vi "readModbusRxData.vi"(8 "error in (no error)":errorcluster, 9 "Timeout (ms)":i32, 10 "ModbusBuffer in":refnum<class "ModbusBuffer.lvclass">, 11 "FPGA in":refnum<class "FPGA.lvclass">) -> (0 "error out":errorcluster, 1 "Elements Remaining":u32, 2 "ModbusBuffer out":refnum<class "ModbusBuffer.lvclass">, 3 "FPGA out":refnum<class "FPGA.lvclass">)   [LabVIEW 2016, in "FPGA.lvclass"]
uses:
  FPGA.lvclass
  Common_RT_Modbus/ModbusBuffer/ModbusBuffer.lvclass
  FPGA.lvclass/FPGA.ctl
  Common_RT_Modbus/ModbusBuffer/ModbusBuffer.lvclass/ModbusBuffer.ctl
  <vilib>/Utility/error.llb/Error Cluster From Error Code.vi
  <vilib>/rvi/errors/niLvFpgaAdjustHostInterfaceError.vi
  <vilib>/rvi/interface/nirviMethod/nirviMethod.xnode
  <vilib>/rvi/errors/niLvFpgaMergeErrorWithErrorCode.vi
  <vilib>/FPGAPlugInAG/Dynamic/niLvFpga_ReadFifo_Dynamic.vi
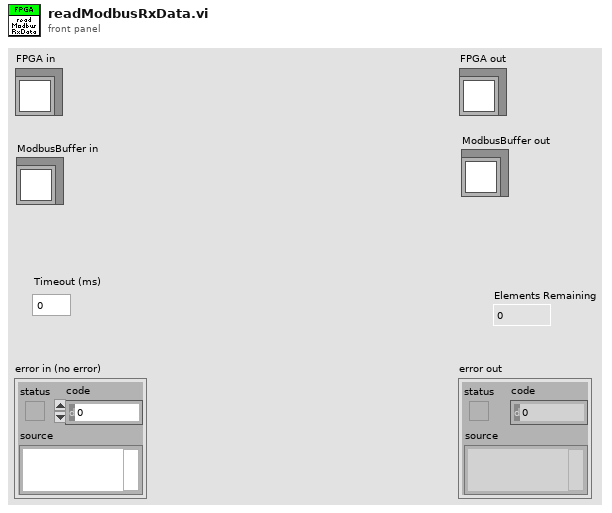
[diagram p1: front panel]
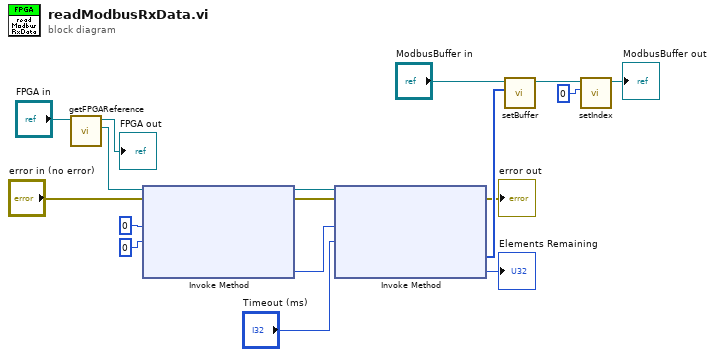
[diagram p0: block diagram]
diagram:
  n1 = call "getFPGAReference.vi"("FPGA in"="FPGA in") -> ("FPGAReference"=w6:refnum<k20>, "FPGA out"=→"FPGA out":refnum<class "FPGA.lvclass">)  [unwired: 9 in]
  n2 = xnode "Invoke Method"("FPGA VI Reference In"=w6, "error in"="error in (no error)", "Number of Elements"=u32 0, "Timeout (ms)"=0) -> ("FPGA VI Reference Out"=w5:refnum<k20>, "error out"=w4:errorcluster, "Elements Remaining"=w13:u32)  [unwired: 1 out]
  n3 = xnode "Invoke Method"("FPGA VI Reference In"=w5, "error in"=w4, "Number of Elements"=w13, "Timeout (ms)"="Timeout (ms)") -> ("error out"=→"error out":errorcluster, "Data"=w8:u16[], "Elements Remaining"=→"Elements Remaining":u32)  [unwired: 1 out]
  n4 = call "setBuffer.vi"("Buffer"=w8, "ModbusBuffer in"="ModbusBuffer in") -> ("ModbusBuffer out"=w11:refnum<class "ModbusBuffer.lvclass">)  [unwired: 9 in]
  n5 = call "setIndex.vi"("Index"=0, "ModbusBuffer in"=w11) -> ("ModbusBuffer out"=→"ModbusBuffer out":refnum<class "ModbusBuffer.lvclass">)  [unwired: 9 in]
